vi "Acquisition Stream Control (IQ 8 SPC).vi"(0 "data in":T2[](array[typedef])=[{"I"=0.0, "Q"=0.0, "overflow"=FALSE}, {"I"=0.0, "Q"=0.0, "overflow"=FALSE}, {"I"=0.0, "Q"=0.0, "overflow"=FALSE}, {"I"=0.0, "Q"=0.0, "overflow"=FALSE}, {"I"=0.0, "Q"=0.0, "overflow"=FALSE}, {"I"=0.0, "Q"=0.0, "overflow"=FALSE}, {"I"=0.0, "Q"=0.0, "overflow"=FALSE}, {"I"=0.0, "Q"=0.0, "overflow"=FALSE}], 1 "input valid":bool, 2 "request state":T1, 3 "num samples":u64, 4 "initial ignore":u64, 7 "ready for output (T)":bool=TRUE, 8 "reset":bool, 9 "start trigger":bool) -> (11 "ready for start":bool, 12 "metadata":u64, 14 "data out":T2[](array[typedef]), 15 "output valid":bool, 16 "actual state":T1, 17 "samples transferred":u64, 19 "acquiring":bool)   [LabVIEW 2018, in "Streaming FPGA.lvlib"]
doc: "<B>General</B>\n\nThis VI controls the signal acquisition data flow with a state machine controller. This enables the control and monitoring of finite and continuous streams of data between nodes using 4-wire handshaking.\n\n<B>Signals</B>\n\nThe stream is controlled by the <B>request state</B>, <B>num samples</B>, <B>initial ignore</B> and <B>start trigger</B> inputs. The stream is monitored by the <B>actual state</B>, <B>ready for start</B>, <B>samples transferred</B> and <B>acquiring</B> outputs. In addition, <b>metadata</b> is available for publishing details about the form/function of the stream.\n\nThe upstream node can provide data on the <B>data in</B> input by setting the <B>input valid</B> input to true. The data provided on the <B>data in</B> input is accepted if the <B>input valid</B> input is true.\n\nThe <B>output valid</B> output is set to true when data is available on the <B>data out</B> output. The downstream node should set the <B>ready for output</B> input to true when it is ready for data. If the <B>ready for output</B> input is true and the <B>output valid</B> output is also true, then the downstream node should accept the data provided on the <B>data out</B> output. If the <B>ready for output</B> input is false or if the <B>output valid</B> output is false, then the downstream should ignore the <B>data out</B> output.\n\nNote that this VI doesn't have a \"ready for input\" output. The data provided by the upstream node is always accepted, but if an acquisition is in progress and the downstream node is not able to accept the data provided by the upstream node, then the acquisition aborts.\n\n<B>Detailed Operation</B>\n\nIf an acquisition is in progress, then the samples provided on the data input are returned on the data output. If no acquisition is in progress then the samples provided on the data input are ignored.\n\nThere are two signal acquisition modes: finite or continuous mode. Each time a signal acquisition is started the controller ignores <B>initial ignore</B> number of input samples, then transfers <B>num samples</B> samples (in case of finite mode) or an unspecified number of samples (in case of continuous mode) from the data input to the data output. A finite signal acquisition can be started by transitioning the state machine from the Idle state to the Finite Transfer state. A continuous signal acquisition can be started by transitioning the state machine from the Idle state to the Continuous state. Transitioning from the Idle state to the Finite Transfer or Continuous state does not start the signal acquisition immediately, when transitioning into these states the state machine always waits for a start trigger before starting the acquisition. The state machine sets the <B>ready for start</B> output to true when it is waiting for a start trigger in the next cycle (otherwise this output is false), the start trigger can be provided on the <B>start trigger</B> input by setting this input to true. The acquisition starts in the cycle when the <B>start trigger</B> input is true and the <B>ready for start</B> output was true in the previous cycle. The data provided on the data input in this cycle is the first data input that is part of the acquisition. The start of the acquisition is also signaled by the <B>acquiring</B> output becoming true. This output is set to false when the acquisition ends. Note that this VI assumes that the signal acquisition should be continuous: during the signal acquisition if the <B>ready for output</B> input is false while data is available on the data output, the state machine aborts the signal acquisition and enters the Error state.\n\n<B>samples transferred</B> is updated with the number of upstream node provided samples accepted by the downstream node in the current cycle, that is, this counter does not include the number of initial samples ignored during the acquisition.\n\nIn finite mode the state machine enters the Done state once the signal acquisition is finished. In the Done state the samples transferred continues to be reported until the user requests that the state machine return to Idle. A signal acquisition can be aborted by entering the Cancel state. When entering the Cancel state, the state machine transitions to the Not Ready state, then it can transition into the Idle state.\n\nIn order to reset this VI set the <B>request state</B> input to Idle, set the <B>reset</B> input to true, wait until the <B>actual state</B> output indicates Idle, then set the <B>reset</B> input to false.\n\n<b>States</b>\n\nThere are seven potential states for a stream defined by the Stream State.ctl typedef. All commanded states should be monitored from the controlling loop if it is important to ensure that the state is actually entered. The <B>request state</B> commands the stream into a state, and <B>actual state</B> reflects the current actual state.\n\nIdle - when the stream is ready to enter into an active state, it is in the Idle state. While it can be commanded directly to Idle from any state, it is advisable to do so with caution as samples abandoned in transfers may still need to be manually cleared out. It is generally safe to go directly from Done to Idle, and it is generally safe to request a transition from Not Ready to Idle. Other states may require further clean-up such as stopping/starting FIFOs or resetting other code under the command of the stream. Consider using Cancel instead (such as through the \"Stop Stream.vi\" in the host environment). While in Idle, <B>samples transferred</B> is reset to 0.\n\nFinite Transfer - Execute a transfer for the requested number of samples. Upon an orderly completion, this VI will automatically enter the Done state. If a stream overflows because the <B>ready for output</B> input is false while data is available on the data output, then the state machine enters the Error state.\n\nContinuous - Execute a transfer indefinitely. This state operates identically to the Finite Transfer state, but without regard to the <B>num samples</B> input.\n\nDone - In an orderly termination of a finite stream, the stream should end up here. At this point, <B>samples transferred</B> accurately reflects the terminal state of the transfer. The Done state should be exited by requesting Idle. Further active transfer modes (Finite or Continuous) will be ignored. This allows the host to distinguish between streams that are prematurely terminated (thus potentially requiring a flush of abandoned data) and ones that completed naturally.\n\nError - If the stream detects an unplanned interruption of the data, it enters the Error state. The only way to exit the Error state is to command the Acquisition Stream Control to Idle or Not Ready. When commanded to Idle or Not Ready, the Acquisition Stream Control advances first to Not Ready.\n\nNot Ready - In this state, the Acquisition Stream Control remains in the Not Ready state until it is commanded to Idle. This prevents starting a transfer in an obviously invalid state, and allows host control to wait until the not ready state is removed (such as by clearing out a FIFO under the streaming API's control).\n\nCancel - This state is indistinguishable from Error, but allows the controlling VI to know what condition caused the transfer to terminate."
uses:
  Streaming FPGA.lvlib
  <instrlib>/_niInstr/DSP/v1/Shared/Public/IQ Data.ctl
  <instrlib>/_niInstr/Streaming/v1/Common/Stream State.ctl
  <instrlib>/_niInstr/DSP/v1/Shared/niInstr DSP v1 Shared.lvlib
  <instrlib>/_niInstr/Streaming/v1/Common/niInstr Streaming v1 Common.lvlib
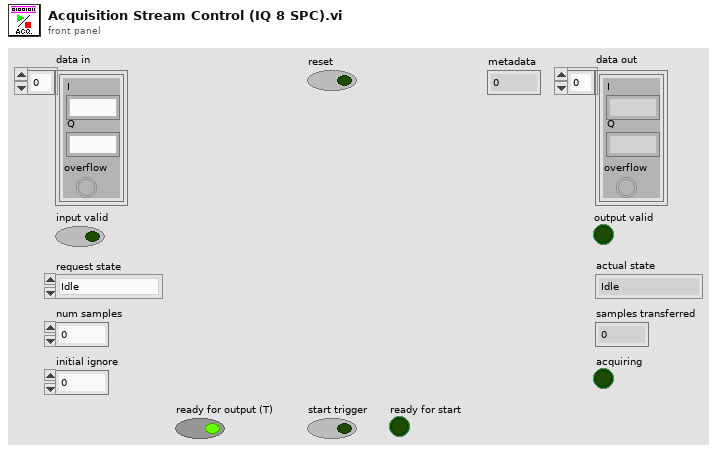
[diagram p1: front panel]
types:
  T1 = typedef "niInstr Streaming v1 Common.lvlib/Stream State.ctl" = enum8{"Idle", "Finite Transfer", "Continuous", "Done", "Error", "Not Ready", "Cancel"}
  T2 = typedef "niInstr DSP v1 Shared.lvlib/IQ Data.ctl" = cluster{"I":fxp<+/-,18,1>, "Q":fxp<+/-,18,1>, "overflow":bool}
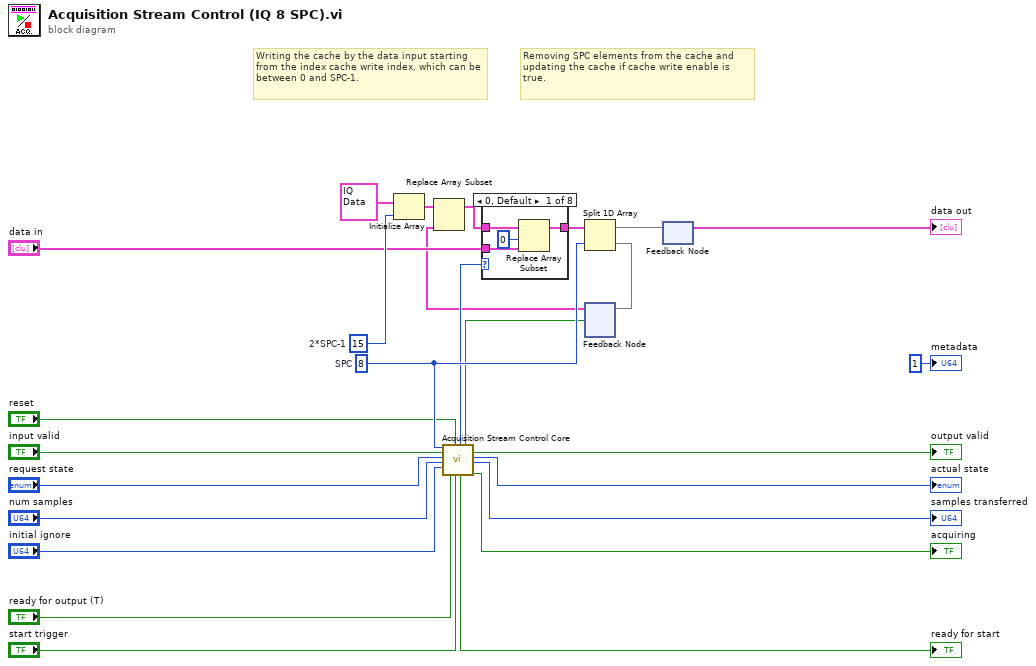
[diagram p0: block diagram]
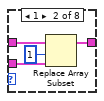
[diagram p2: hidden frame]
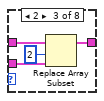
[diagram p3: hidden frame]
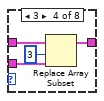
[diagram p4: hidden frame]
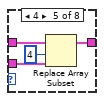
[diagram p5: hidden frame]
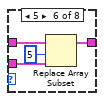
[diagram p6: hidden frame]
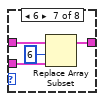
[diagram p7: hidden frame]
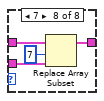
[diagram p8: hidden frame]
diagram:
  w21 = u8 8  # SPC
  w26 = u8 15  # 2*SPC-1
  # "Removing SPC elements from the cache and updating the cache if cache write enable is true."
  # "Writing the cache by the data input starting from the index cache write index, which can be between 0 and SPC-1."
  n1 = Initialize Array(T2 {"I"=0.0, "Q"=0.0, "overflow"=FALSE}, w26) -> (w7:T2[])
  n2 = call "Acquisition Stream Control Core.vi"("SPC"=w21, "input valid"="input valid", "request state"="request state", "num samples"="num samples", "initial ignore"="initial ignore", "ready for output (T)"="ready for output (T)", "reset"="reset", "start trigger"="start trigger") -> ("cache write index"=w9:u8, "ready for start"=→"ready for start":bool, "cache write enable"=w8:bool, "output valid"=→"output valid":bool, "actual state"=→"actual state":T1, "samples transferred"=→"samples transferred":u64, "acquiring"=→"acquiring":bool)  [unwired: 5 in]
  n3 = feedback #1() -> (w5:T2[])  [unwired: 1 in]
  n4 = Replace Array Subset(array=w7, new element=w5) -> (w6:T2[])  [unwired: 1 in]
  n5 = case shown="0, Default" w9 {
    tunnel: w6 -> [w30 w34 w38 w42 w46 w50 w54 w58]
    tunnel: "data in" -> [w29 w33 w37 w41 w45 w49 w53 w57]
    tunnel: [w27 w31 w35 w39 w43 w47 w51 w55] -> w23
    frame 0, Default {
      n6 = Replace Array Subset(array=w30, new element=w29, index=0) -> (w27:T2[])
    }
    frame 1 {
      n7 = Replace Array Subset(array=w34, new element=w33, index=1) -> (w31:T2[])
    }
    frame 2 {
      n8 = Replace Array Subset(array=w38, new element=w37, index=2) -> (w35:T2[])
    }
    frame 3 {
      n9 = Replace Array Subset(array=w42, new element=w41, index=3) -> (w39:T2[])
    }
    frame 4 {
      n10 = Replace Array Subset(array=w46, new element=w45, index=4) -> (w43:T2[])
    }
    frame 5 {
      n11 = Replace Array Subset(array=w50, new element=w49, index=5) -> (w47:T2[])
    }
    frame 6 {
      n12 = Replace Array Subset(array=w54, new element=w53, index=6) -> (w51:T2[])
    }
    frame 7 {
      n13 = Replace Array Subset(array=w58, new element=w57, index=7) -> (w55:T2[])
    }
  }
  n14 = Split 1D Array(array=w23, index=w21) -> (first subarray=w22:T2[], second subarray=w4:T2[])
  n15 = feedback-in #1(w4, w8) -> ()
  n16 = feedback-in #2(w22) -> ()
  n17 = feedback #2() -> (→"data out":T2[])  [unwired: 1 in]
  "metadata" <- u64 1 ("metadata")
